vi "Get Params.vi"(8 "error in (no error)":errorcluster, 10 "Log Class":refnum<class "Build_Javier_Lopez_lib_Configuration_Filejson class.lvclass">, 11 "Module Com in":refnum<class "Communication.lvclass">) -> (0 "error out":errorcluster, 3 "Module Com out":refnum<class "Communication.lvclass">)   [LabVIEW 2021, in "Communication.lvclass"]
uses:
  Communication.lvclass
  <vilib>/Javier Lopez/Configuration File/Json Element/Build_Javier_Lopez_lib_Configuration_Filejson class.lvclass
  Communication.lvclass/Communication.ctl
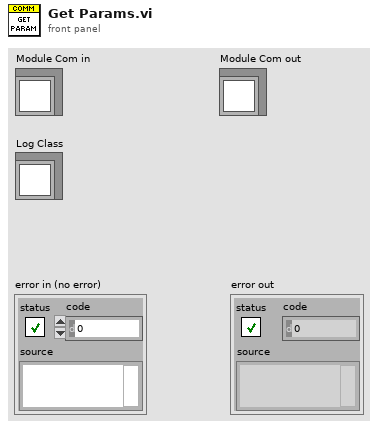
[diagram p1: front panel]
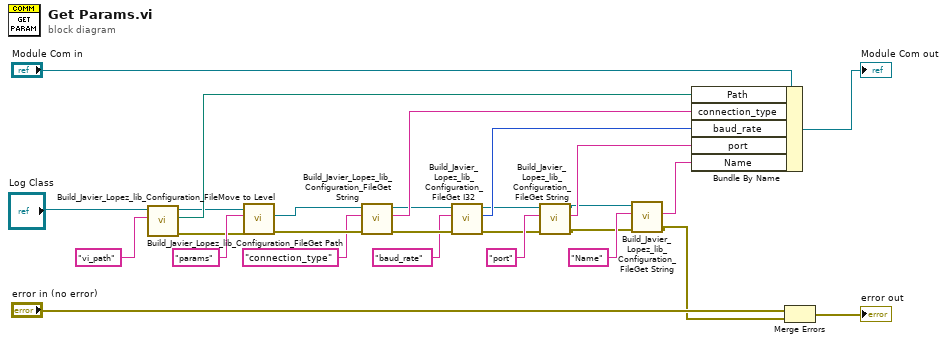
[diagram p0: block diagram]
diagram:
  n1 = call <vilib>:"Build_Javier_Lopez_lib_Configuration_FileGet Path.vi"("Name"="vi_path", "json class in"="Log Class") -> ("error out"=w2:errorcluster, "Path"=w24:path, "json class out"=w21:refnum<class "Build_Javier_Lopez_lib_Configuration_Filejson class.lvclass">)  [unwired: 7 in]
  n2 = call-dynamic "Build_Javier_Lopez_lib_Configuration_FileMove to Level.vi"("error in (no error)"=w2, "Element"="params" ("Name"), "json class in"=w21) -> ("error out"=w19:errorcluster, "New json class"=w18:refnum<class "Build_Javier_Lopez_lib_Configuration_Filejson class.lvclass">)  [unwired: 6 in, 1 out]
  n3 = call <vilib>:"Build_Javier_Lopez_lib_Configuration_FileGet String.vi"("error in (no error)"=w19, "Name"="connection_type", "json class in"=w18) -> ("error out"=w14:errorcluster, "String"=w16:string, "json class out"=w15:refnum<class "Build_Javier_Lopez_lib_Configuration_Filejson class.lvclass">)  [unwired: 6 in]
  n4 = call <vilib>:"Build_Javier_Lopez_lib_Configuration_FileGet I32.vi"("error in (no error)"=w14, "Name"="baud_rate", "json class in"=w15) -> ("error out"=w5:errorcluster, "I32"=w12:i32, "json class out"=w6:refnum<class "Build_Javier_Lopez_lib_Configuration_Filejson class.lvclass">)  [unwired: 6 in]
  n5 = call <vilib>:"Build_Javier_Lopez_lib_Configuration_FileGet String.vi"("error in (no error)"=w5, "Name"="port", "json class in"=w6) -> ("error out"=w4:errorcluster, "String"=w8:string, "json class out"=w7:refnum<class "Build_Javier_Lopez_lib_Configuration_Filejson class.lvclass">)  [unwired: 6 in]
  n6 = call <vilib>:"Build_Javier_Lopez_lib_Configuration_FileGet String.vi"("error in (no error)"=w4, "Name"="Name", "json class in"=w7) -> ("error out"=w3:errorcluster, "String"=w9:string)  [unwired: 6 in, 1 out]
  n7 = Bundle By Name(cluster="Module Com in", "Path"=w24, "connection_type"=w16, "baud_rate"=w12, "port"=w8, "Name"=w9) -> (→"Module Com out":refnum<class "Communication.lvclass">)
  n8 = Merge Errors("error in (no error)", w3) -> (→"error out":errorcluster)
